vi "MT Detect QAM.vi"(5 "input complex waveform":T3={"t0"=0.0, "dt"=1.0, "Y"=[]} {"Y" format="%.3f"; "dt" format="%^.2e"; "t0" format="%.4f"}, 7 "QAM system parameters":T2={"samples per symbol (16)"=16, "symbol map"=[]} {"symbol map" format="%.3f"}, 9 "synchronization parameters":T1 {"sync sequence" format="%.2f"}, 11 "error in (no error)":errorcluster, 12 "matched filter coefficients":dbl[](array[numeric]) format="%.2f", 13 "reset? (T)":bool=TRUE, 14 "flush buffers? (F)":bool) -> (6 "output bit stream":i8[](array[numeric]), 10 "sync found index (symbols)":dbl format="%.4f", 15 "error out":errorcluster)   [LabVIEW 2020, in "niDMT.lvlib"]
doc: "Demodulates a quadrature-amplitude modulation (QAM)-modulated complex baseband waveform and returns the demodulated bit stream. This VI attempts to remove carrier and phase offset by locking to the carrier signal."
uses:
  <vilib>/addons/Modulation/niDMT.lvlib
  <vilib>/addons/Modulation/Analog/controls/Complex Data Waveform.ctl
  <vilib>/Utility/error.llb/Error Cluster From Error Code.vi
  <vilib>/addons/Modulation/Digital/Support/Common/mod_Truncate FIR Filter (complex).vi
  <vilib>/addons/Modulation/niAMT.lvlib
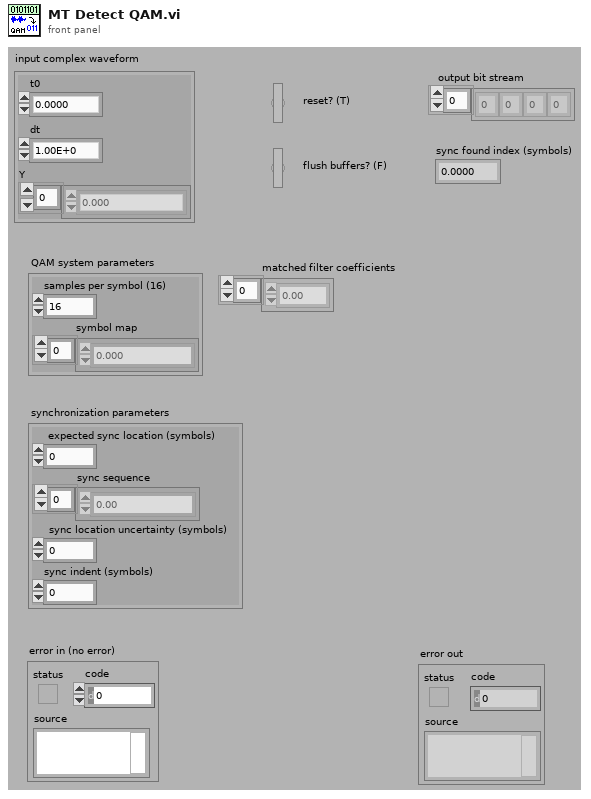
[diagram p1: front panel]
types:
  T1 = cluster{"expected sync location (symbols)":i32, "sync sequence":cdb[], "sync location uncertainty (symbols)":i32, "sync indent (symbols)":i32}
  T2 = cluster{"samples per symbol (16)":i32, "symbol map":cdb[]}
  T3 = typedef "niAMT.lvlib/Complex Data Waveform.ctl" = cluster{"t0":dbl, "dt":dbl, "Y":cdb[]}
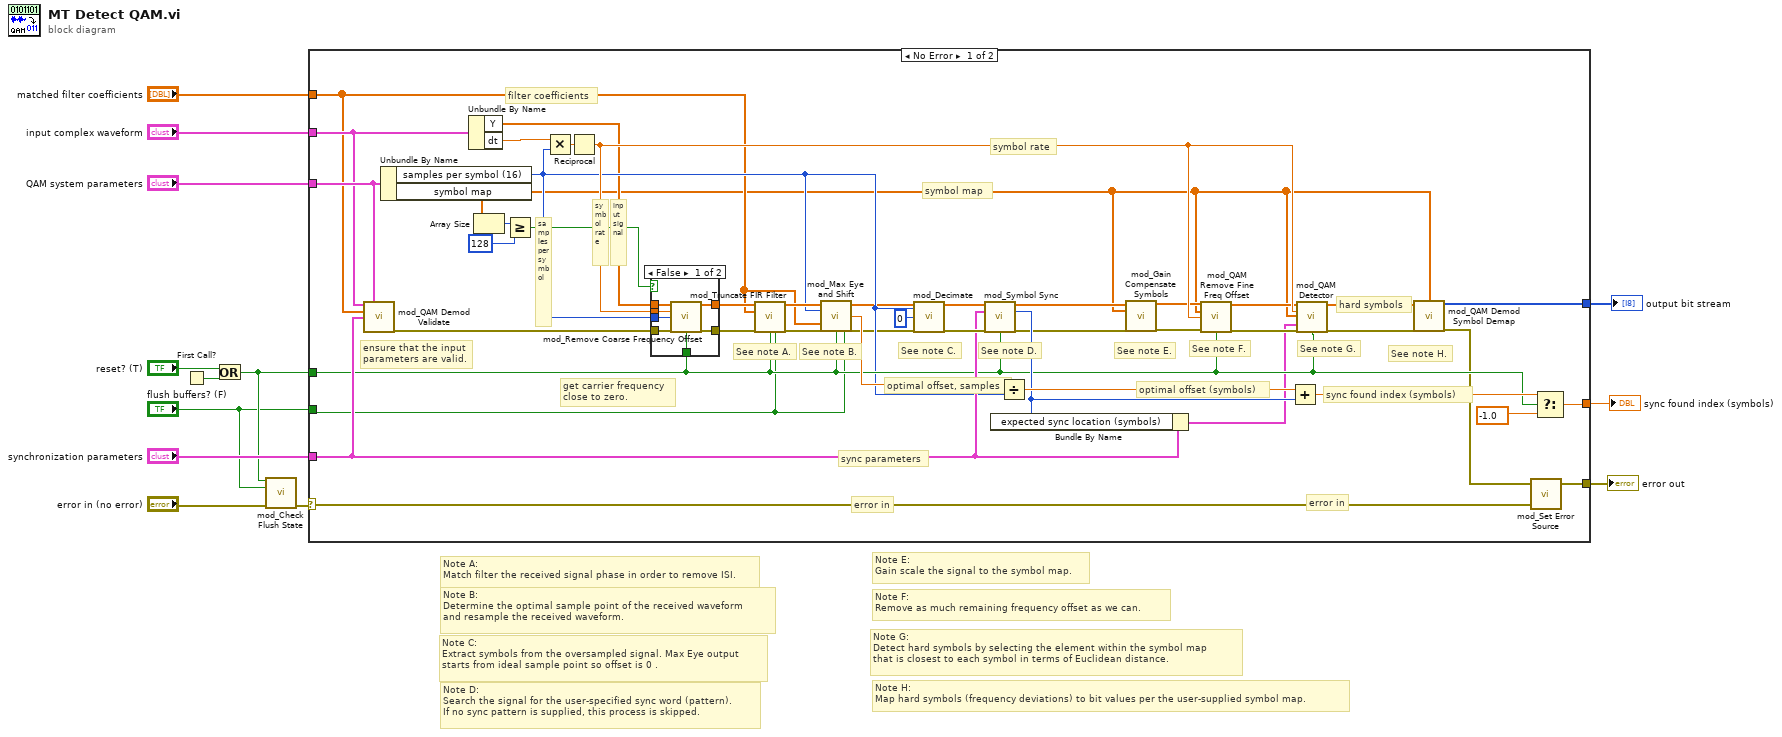
[diagram p0: block diagram]
diagram:
  # "Note E:\nGain scale the signal to the symbol map."
  # "Note H:\nMap hard symbols (frequency deviations) to bit values per the user-supplied symbol map."
  # "Note D:\nSearch the signal for the user-specified sync word (pattern). \nIf no sync pattern is supplied, this process is skipped."
  # "Note F:\nRemove as much remaining frequency offset as we can."
  # "Note C:\nExtract symbols from the oversampled signal. Max Eye output\nstarts from ideal sample point so offset is 0 ."
  # "Note B:\nDetermine the optimal sample point of the received waveform \nand resample the received waveform."
  # "Note A:\nMatch filter the received signal phase in order to remove ISI."
  # "Note G:\nDetect hard symbols by selecting the element within the symbol map \nthat is closest to each symbol in terms of Euclidean distance."
  n1 = First Call?() -> (First Call?: T/F=w6:bool)
  n2 = Or(x="reset? (T)", y=w6) -> (x .or. y?=w3:bool)
  n3 = call <vilib>:"mod_Check Flush State.vi"("reset?"=w3, "flush buffers? (F)"="flush buffers? (F)", "error in (no error)"="error in (no error)") -> ("error out"=w4:errorcluster)  [unwired: 12 out]
  n4 = case shown="No Error" w4 {
    selector: w4 -> [w32 w67]
    tunnel: w3 -> [w36 _]
    tunnel: "input complex waveform" -> [w42 _]
    tunnel: [w31 w67] -> w7
    tunnel: "matched filter coefficients" -> [w22 _]
    tunnel: [w57 _] -> w9
    tunnel: [w43 _] -> w8
    tunnel: "QAM system parameters" -> [w55 _]
    tunnel: "synchronization parameters" -> [w48 _]
    tunnel: "flush buffers? (F)" -> [w19 _]
    frame No Error {
      # "filter coefficients"
      # "See note G."
      # "error in"
      # "sync found index (symbols)"
      # "symbol rate"
      # "hard symbols"
      # "sync parameters"
      # "error in"
      # "symbol map"
      # "samples per symbol"
      # "input signal"
      # "See note E."
      # "See note H."
      # "See note D."
      # "See note F."
      # "See note C."
      # "get carrier frequency close to zero."
      # "ensure that the input parameters are valid."
      # "See note B."
      # "See note A."
      # "optimal offset (symbols)"
      # "optimal offset, samples"
      # "symbol rate"
      n5 = call <vilib>:"mod_QAM Demod Validate.vi"("Input Complex Waveform"=w42, "QAM System Parameters"=w55, "Matched Filter Coefficients"=w22, "Synchronization Parameters"=w48) -> ("error out"=w50:errorcluster)  [unwired: 11 out]
      n6 = Unbundle By Name(w55) -> ("samples per symbol (16)"=w34:i32, "symbol map"=w17:cdb[])
      n7 = Unbundle By Name(w42) -> ("Y"=w20:cdb[], "dt"=w21:dbl)
      n8 = Array Size(array=w17) -> (size(s)=w14:i32)
      n9 = Greater Or Equal?(x=w14, y=128) -> (x >= y?=w15:bool)
      n10 = Multiply(x=w21, y=w34) -> (x*y=w53:dbl)
      n11 = Reciprocal(x=w53) -> (1/x=w49:dbl)
      n12 = case shown="False" w15 {
        tunnel: [w64 w65] -> w56
        tunnel: w50 -> [w63 w65]
        tunnel: w49 -> [w62 _]
        tunnel: [w61 w66] -> w39
        tunnel: w36 -> [w60 _]
        tunnel: w34 -> [w59 _]
        tunnel: w20 -> [w58 w66]
        frame False {
          n13 = call <vilib>:"mod_Remove Coarse Frequency Offset.vi"("Signal In"=w58, "Symbol Rate, Hz"=w62, "Samples Per Symbol (16)"=w59, "error in (no error)"=w63, "Reset? (T)"=w60) -> ("Signal Out"=w61:cdb[], "error out"=w64:errorcluster)  [unwired: 3 in, 6 out]
        }
        frame True {
        }
      }
      n14 = call-poly <vilib>:"mod_Truncate FIR Filter.vi"("Signal In"=w39, "Filter Coefficients"=w22, "error in (no error)"=w56, "Reset? (T)"=w36, "flush buffers? (F)"=w19) -> ("Signal Out"=w38:cdb[], "error out"=w51:errorcluster)  [unwired: 9 out]
      n15 = call <vilib>:"mod_Max Eye and Shift.vi"("Signal In"=w38, "Samples Per Symbol (16)"=w34, "matched filter coefficients"=w22, "error in (no error)"=w51, "Reset? (T)"=w36, "flush buffers? (F)"=w19) -> ("Signal Out"=w24:cdb[], "Optimal Offset (in Samples)"=w40:dbl, "error out"=w23:errorcluster)  [unwired: 7 out]
      n16 = call <vilib>:"mod_Decimate.vi"("Signal In"=w24, "Samples Per Symbol (16)"=w34, "Offset"=0, "error in (no error)"=w23) -> ("Signal Out"=w35:cdb[], "error out"=w54:errorcluster)  [unwired: 1 in, 9 out]
      n17 = call <vilib>:"mod_Symbol Sync.vi"("Signal In"=w35, "Synchronization Parameters"=w48, "error in (no error)"=w54, "Reset? (T)"=w36) -> ("Signal Out"=w28:cdb[], "Sync Location (symbols)"=w47:i32, "error out"=w30:errorcluster)  [unwired: 1 in, 8 out]
      n18 = Bundle By Name(cluster=w48, "expected sync location (symbols)"=w47) -> (w18:T1)
      n19 = Divide(x=w40, y=w34) -> (x/y=w52:dbl)
      n20 = call <vilib>:"mod_Gain Compensate Symbols.vi"("Symbols In"=w28, "Symbol Map"=w17, "error in (no error)"=w30) -> ("Symbols Out"=w27:cdb[], "error out"=w29:errorcluster)  [unwired: 1 in, 10 out]
      n21 = call <vilib>:"mod_QAM Remove Fine Freq Offset.vi"("Symbols"=w27, "Symbol Map"=w17, "Symbol Rate, Hz"=w49, "error in (no error)"=w29, "Reset? (T)"=w36) -> ("Symbols"=w41:cdb[], "error out"=w46:errorcluster)  [unwired: 9 out]
      n22 = Add(x=w52, y=w47) -> (x+y=w44:dbl)
      n23 = call <vilib>:"mod_QAM Detector.vi"("Signal In"=w41, "Symbol Rate, Hz"=w49, "Symbol Map"=w17, "Synchronization Parameters"=w18, "error in (no error)"=w46, "Reset? (T)"=w36) -> ("Signal Out"=w26:cdb[], "error out"=w25:errorcluster)  [unwired: 2 in, 6 out]
      n24 = call <vilib>:"mod_QAM Demod Symbol Demap.vi"("Symbols In"=w26, "Symbol Map"=w17, "error in (no error)"=w25) -> ("Bits Out"=w57:i8[], "error out"=w33:errorcluster)  [unwired: 1 in, 10 out]
      n25 = call <vilib>:"mod_Set Error Source.vi"("initial error in (no error)"=w32, "final error in (no error)"=w33) -> ("error out"=w31:errorcluster)  [unwired: 3 out]
      n26 = Select(t=w44, s=w36, f=-1.0) -> (s? t:f=w43:dbl)
    }
    frame Error {
    }
  }
  "error out" <- w7
  "sync found index (symbols)" <- w8
  "output bit stream" <- w9
